vi "OnCommandLine Event Callback.vi"(4 "Command Line Message":refnum<user-event>, 5 "Event Data":cluster{"seconds":dbl, "cmdLine":string}, 6 "Control Ref":refnum<k24>, 7 "Event Common Data":T1) -> ()   [LabVIEW 2020, in "NI_VS MacroRecorderAPI.lvlib"]
uses:
  <vilib>/NI VeriStand/Execution/MacroRecorder/NI_VS MacroRecorderAPI.lvlib
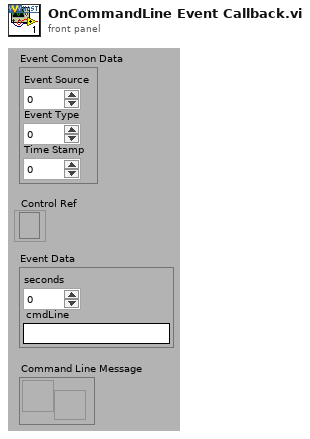
[diagram p1: front panel]
types:
  T1 = cluster{"Event Source":i32, "Event Type":u32, "Time Stamp":u32}
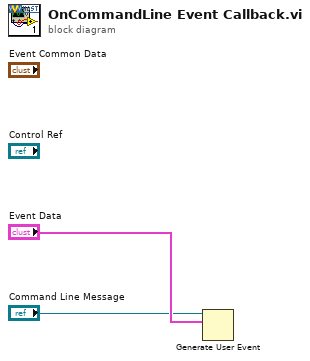
[diagram p0: block diagram]
diagram:
  n1 = Generate User Event(user event="Command Line Message", event data cluster="Event Data") -> ()  [unwired: 2 in, 2 out]
